vi "test DSF Reentrancy.vi"(8 "error in (no error)":errorcluster, 11 "TestCase in":refnum<class "Reentrancy Tests.lvclass">) -> (0 "error out":errorcluster, 3 "TestCase out":refnum<class "Reentrancy Tests.lvclass">)   [LabVIEW 2019, in "Reentrancy Tests.lvclass"]
uses:
  Reentrancy Tests.lvclass
  <vilib>/addons/_JKI Toolkits/VI Tester/TestCase.llb/TestCase.lvclass
  C:/Program Files (x86)/National Instruments/LabVIEW 2019/vi.lib/addons/_JKI Toolkits/VI Tester/TestCase.llb/TestCase.lvclass
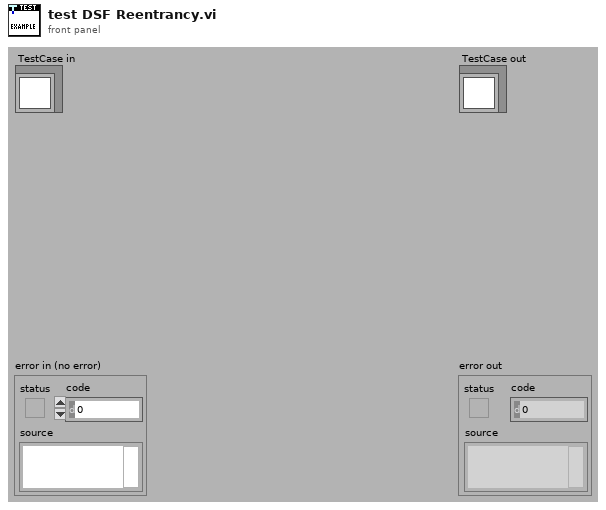
[diagram p1: front panel]
types:
  T1 = enum16{"Indices (0, 2, 4, ...)", "Indices (1, 3, 5, ...)", "All"}
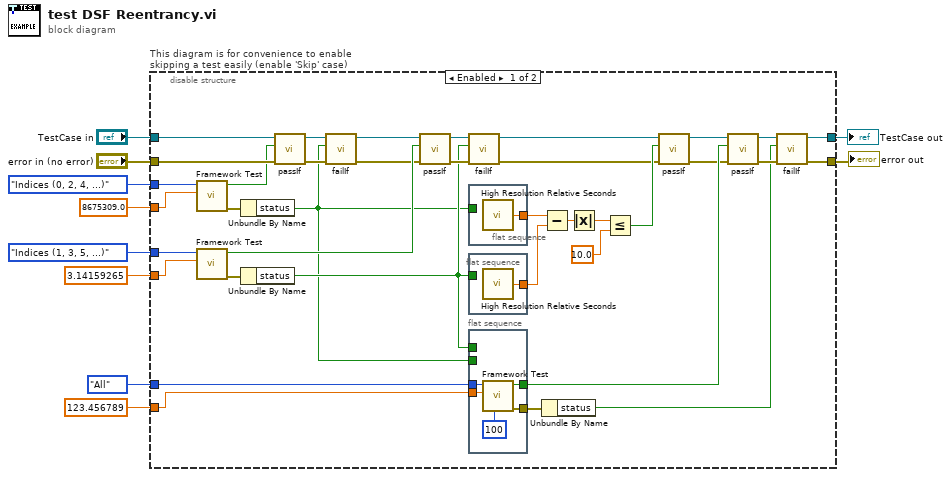
[diagram p0: block diagram]
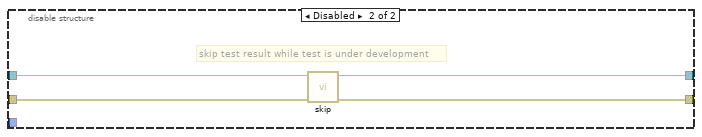
[diagram p2: hidden frame]
diagram:
  n1 = disable-structure "This diagram is for convenience to enable skipping a test easily (enable 'Skip' case)" shown="Enabled" {
    disable-tunnel: "TestCase in" -> [w47 w58]
    disable-tunnel: [w17 w56] -> w7
    disable-tunnel: [w16 w57] -> w9
    disable-tunnel: "error in (no error)" -> [w46 w55]
    disable-tunnel: T1."All" ("channel selection") -> [w30 _]
    disable-tunnel: T1."Indices (1, 3, 5, ...)" ("channel selection") -> [w29 _]
    disable-tunnel: T1."Indices (0, 2, 4, ...)" ("channel selection") -> [w28 _]
    disable-tunnel: 8675309.0 ("channel values") -> [w13 _]
    disable-tunnel: 3.14159265 ("channel values") -> [w12 _]
    disable-tunnel: 123.456789 ("channel values") -> [w11 _]
    frame Enabled {
      n2 = call "Framework Test.vi"("channel values"=w13, "channel selection"=w28) -> ("error out"=w37:errorcluster, "read = write"=w45:bool)  [unwired: 8 in]
      n3 = call "Framework Test.vi"("channel values"=w12, "channel selection"=w29) -> ("error out"=w36:errorcluster, "read = write"=w44:bool)  [unwired: 8 in]
      n4 = Unbundle By Name(w37) -> ("status"=w14:bool)
      n5 = Unbundle By Name(w36) -> ("status"=w15:bool)
      n6 = call-dynamic "passIf.vi"("error in (no error)"=w46, "pass"=w45, "TestCase in"=w47) -> ("error out"=w42:errorcluster, "TestCase out"=w43:refnum<class "Reentrancy Tests.lvclass">)  [unwired: 7 in]
      n7 = call-dynamic "failIf.vi"("error in (no error)"=w42, "fail"=w14, "TestCase in"=w43) -> ("error out"=w40:errorcluster, "TestCase out"=w41:refnum<class "Reentrancy Tests.lvclass">)  [unwired: 7 in]
      n8 = call-dynamic "passIf.vi"("error in (no error)"=w40, "pass"=w44, "TestCase in"=w41) -> ("error out"=w38:errorcluster, "TestCase out"=w39:refnum<class "Reentrancy Tests.lvclass">)  [unwired: 7 in]
      n9 = call-dynamic "failIf.vi"("error in (no error)"=w38, "fail"=w15, "TestCase in"=w39) -> ("error out"=w20:errorcluster, "TestCase out"=w21:refnum<class "Reentrancy Tests.lvclass">)  [unwired: 7 in]
      n10 = flat-sequence {
        tunnel: w14 -> [_]
        tunnel: [w54] -> w35
        frame #0 {
          n11 = call <vilib>:"High Resolution Relative Seconds.vi"() -> ("relative seconds"=w54:dbl)
        }
      }
      n12 = flat-sequence {
        tunnel: w15 -> [_]
        tunnel: [w53] -> w27
        frame #0 {
          n13 = call <vilib>:"High Resolution Relative Seconds.vi"() -> ("relative seconds"=w53:dbl)
        }
      }
      n14 = flat-sequence {
        tunnel: [w52] -> w31
        tunnel: w30 -> [w51]
        tunnel: [w50] -> w22
        tunnel: w15 -> [_]
        tunnel: w14 -> [_]
        tunnel: w11 -> [w48]
        frame #0 {
          n15 = call "Framework Test.vi"("max iterations"=u64 100, "channel values"=w48, "channel selection"=w51) -> ("error out"=w52:errorcluster, "read = write"=w50:bool)  [unwired: 7 in]
        }
      }
      n16 = Subtract(x=w35, y=w27) -> (x-y=w34:dbl)
      n17 = Unbundle By Name(w31) -> ("status"=w23:bool)
      n18 = Absolute Value(x=w34) -> (abs(x)=w33:dbl)
      n19 = Less Or Equal?(x=w33, y=10.0) -> (x <= y?=w32:bool)
      n20 = call-dynamic "passIf.vi"("error in (no error)"=w20, "pass"=w32, "TestCase in"=w21) -> ("error out"=w18:errorcluster, "TestCase out"=w19:refnum<class "Reentrancy Tests.lvclass">)  [unwired: 7 in]
      n21 = call-dynamic "passIf.vi"("error in (no error)"=w18, "pass"=w22, "TestCase in"=w19) -> ("error out"=w25:errorcluster, "TestCase out"=w24:refnum<class "Reentrancy Tests.lvclass">)  [unwired: 7 in]
      n22 = call-dynamic "failIf.vi"("error in (no error)"=w25, "fail"=w23, "TestCase in"=w24) -> ("error out"=w16:errorcluster, "TestCase out"=w17:refnum<class "Reentrancy Tests.lvclass">)  [unwired: 7 in]
    }
    frame Disabled {
      # "skip test result while test is under development"
      n23 = call <vilib>:"skip.vi"("error in (no error)"=w55, "TestCase in"=w58) -> ("error out"=w57:errorcluster, "TestCase out"=w56:refnum<class "Reentrancy Tests.lvclass">)  [unwired: 8 in]
    }
  }
  "error out" <- w9
  "TestCase out" <- w7
